vi "SemicolonRemover.vi"(3 "output type":enum16{"string", "int", "float"}(ring), 4 "index":i32=5, 5 "Strings":string[](array[string])) -> (0 "float array":dbl[](array[numeric]), 1 "int array":i32[](array[numeric]), 2 "string array":string[](array[string]))   [LabVIEW 2013]
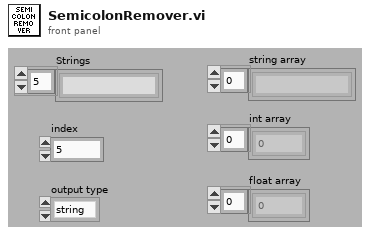
[diagram p1: front panel]
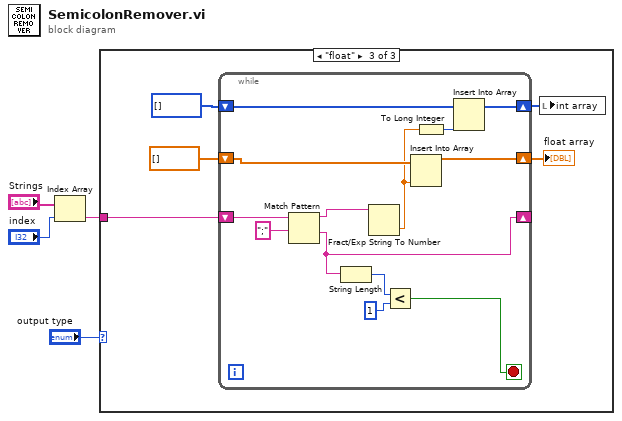
[diagram p0: block diagram]
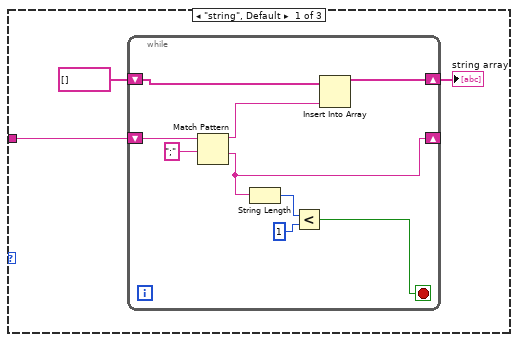
[diagram p2: hidden frame]
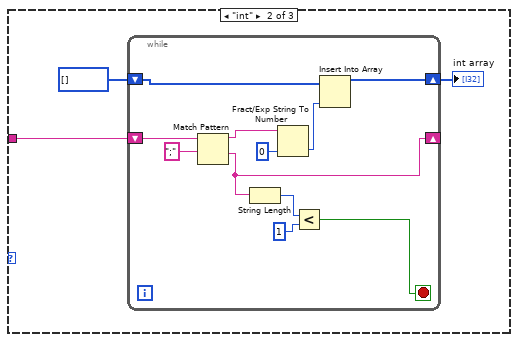
[diagram p3: hidden frame]
diagram:
  n1 = Index Array(array="Strings", index="index") -> (element=w1:string)
  n2 = case shown="\"float\"" "output type" {
    tunnel: w1 -> [w6 w18 w34]
    frame "string", Default {
      n3 = while {
        shift-right: [w10] -> w5
        shift-left: string[] [] -> [w11]
        shift-right: [w9] -> _
        shift-left: w6 -> [w16]
        stop <- w12 stop-if-true
        n4 = Match Pattern(string=w16, regular expression=";") -> (before substring=w8:string, after substring=w9:string)  [unwired: 1 in, 2 out]
        n5 = String Length(string=w9) -> (length=w14:i32)
        n6 = Less?(x=w14, y=1) -> (x < y?=w12:bool)
        n7 = Insert Into Array(array=w11, new element=w8) -> (w10:string[])  [unwired: 1 in]
      }
      "string array" <- w5
    }
    frame "int" {
      n8 = while {
        shift-right: [w23] -> w17
        shift-left: i32[] [] -> [w24]
        shift-right: [w21] -> _
        shift-left: w18 -> [w30]
        stop <- w25 stop-if-true
        n9 = Match Pattern(string=w30, regular expression=";") -> (before substring=w28:string, after substring=w21:string)  [unwired: 1 in, 2 out]
        n10 = String Length(string=w21) -> (length=w27:i32)
        n11 = Fract/Exp String To Number(string=w28, default (0 dbl)=0 ("default (0 DBL)")) -> (number=w22:i32)  [unwired: 2 in, 1 out]
        n12 = Less?(x=w27, y=1) -> (x < y?=w25:bool)
        n13 = Insert Into Array(array=w24, new element=w22) -> (w23:i32[])  [unwired: 1 in]
      }
      "int array" <- w17
    }
    frame "float" {
      n14 = while {
        shift-right: [w41] -> w33
        shift-left: dbl[] [] -> [w42]
        shift-right: [w40] -> _
        shift-left: w34 -> [w48]
        shift-right: [w38] -> w31
        shift-left: i32[] [] -> [w39]
        stop <- w43 stop-if-true
        n15 = Match Pattern(string=w48, regular expression=";") -> (before substring=w46:string, after substring=w40:string)  [unwired: 1 in, 2 out]
        n16 = String Length(string=w40) -> (length=w45:i32)
        n17 = Fract/Exp String To Number(string=w46) -> (number=w36:dbl)  [unwired: 3 in, 1 out]
        n18 = Less?(x=w45, y=1) -> (x < y?=w43:bool)
        n19 = Insert Into Array(array=w42, new element=w36) -> (w41:dbl[])  [unwired: 1 in]
        n20 = To Long Integer(number=w36) -> (32bit integer=w37:i32)
        n21 = Insert Into Array(array=w39, new element=w37) -> (w38:i32[])  [unwired: 1 in]
      }
      "float array" <- w33
      n22 = local write "int array"(w31) -> ()
    }
  }
